vi "StringProbe.vi"(11 "?":string) -> (2 "Value String":string, 3 "Boolean":bool)   [LabVIEW 2017]
doc: "A probe for string data. This probe resizes in the Probe Watch Window."
panel:
  out "Display":string
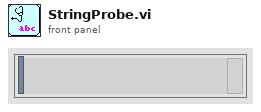
[diagram p1: front panel]
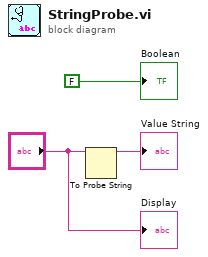
[diagram p0: block diagram]
diagram:
  n1 = To Probe String(7:"?") -> (3:→"Value String":string)  [unwired: 2 in, 1 out]
  "Boolean" <- FALSE ("Boolean")
  "Display" <- "?"
